vi "update.start_time.vi"(8 "error in (no error)":errorcluster, 10 "Start Time (now)":timestamp format="%<%x %.3X>T", 11 "Run in":refnum<class "Run.lvclass">) -> (0 "error out":errorcluster, 3 "Run out":refnum<class "Run.lvclass">)   [LabVIEW 2020, in "Run.lvclass"]
uses:
  Run.lvclass
  Nominal Client/Nominal Client.lvclass
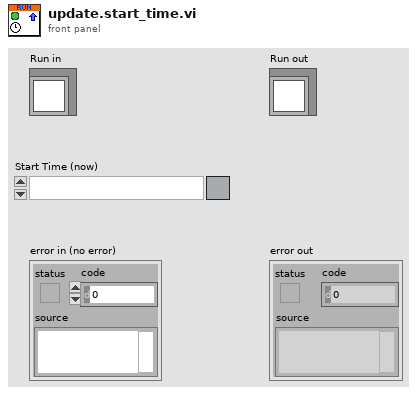
[diagram p1: front panel]
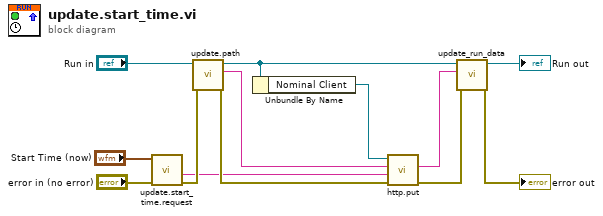
[diagram p0: block diagram]
diagram:
  n1 = call "update.start_time.request.vi"("error in"="error in (no error)", "start time"="Start Time (now)") -> ("error out"=w5:errorcluster, "Request"=w3:string)  [unwired: 8 in]
  n2 = call "update.path.vi"("error in"=w5, "Run"="Run in") -> ("error out"=w4:errorcluster, "path"=w12:string, "Run Out"=w10:refnum<class "Run.lvclass">)  [unwired: 7 in]
  n3 = Unbundle By Name(w10) -> ("Nominal Client"=w11:refnum<class "Nominal Client.lvclass">)
  n4 = call "http.put.vi"("error in"=w4, "Body"=w3, "Path"=w12, "Nominal Client in"=w11) -> ("error out"=w6:errorcluster, "Response"=w9:string)  [unwired: 5 in, 1 out]
  n5 = call "update_run_data.vi"("error in"=w6, "Run JSON"=w9, "Run in"=w10) -> ("error out"=→"error out":errorcluster, "Run out"=→"Run out":refnum<class "Run.lvclass">)  [unwired: 7 in]
